vi "MdfSetHead.vi"(8 "error in (no error)":errorcluster, 11 "MDFRef":refnum<k24>) -> (0 "error IO":errorcluster, 3 "MDFRef out":refnum<k24>)   [LabVIEW 2025, in "MdfFile.lvlib"]
uses:
  MdfFile.lvlib
  data/mdflibrary.dll
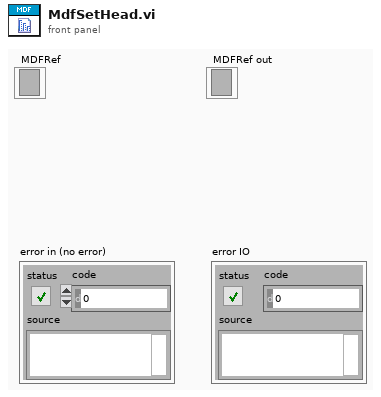
[diagram p1: front panel]
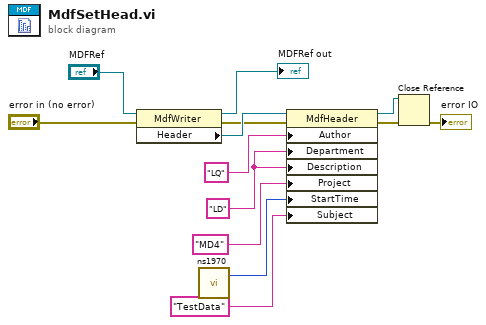
[diagram p0: block diagram]
diagram:
  w8 = "LD" ("Department")
  n1 = property class="MdfWriter"(reference="MDFRef", error in="error in (no error)") -> (reference out=→"MDFRef out":refnum<k24>, error out=w5:errorcluster, "Header"=w13:refnum<k24>)
  n2 = call "ns1970.vi"() -> ("ns1970"=w4:u64)  [unwired: 3 in]
  n3 = property class="MdfHeader"(reference=w13, error in=w5, "Author"="LQ", "Department"=w8, "Description"=w8, "Project"="MD4", "StartTime"=w4, "Subject"="TestData") -> (reference out=w11:refnum<k24>, error out=w10:errorcluster)
  n4 = Close Reference(reference=w11, error in (no error)=w10) -> (error out=→"error IO":errorcluster)
